vi "trigger test.vi"   [LabVIEW 2012]
uses:
  <vilib>/DAQmx/create/channels.llb/DAQmx Create Channel (AI-Voltage-Basic).vi
  <vilib>/DAQmx/configure/timing.llb/DAQmx Timing (Sample Clock).vi
  <vilib>/DAQmx/configure/trigger.llb/DAQmx Start Trigger (Digital Edge).vi
  <vilib>/DAQmx/write.llb/DAQmx Write (Analog 1D Wfm NChan NSamp).vi
  <vilib>/DAQmx/read.llb/DAQmx Read (Analog 1D DBL 1Chan NSamp).vi
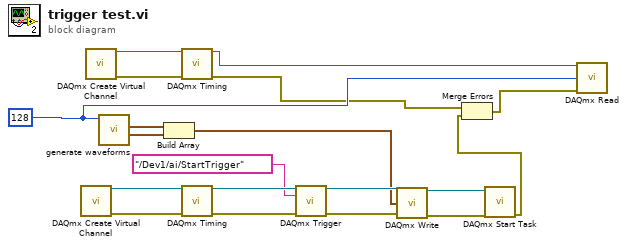
[diagram p0: block diagram]
diagram:
  w6 = 128 ("Number of Samples")
  n1 = call-poly <vilib>:"DAQmx Create Virtual Channel.vi"() -> ("task out"=w18:refnum<k21>, "error out"=w19:errorcluster)  [unwired: 14 in]
  n2 = call-poly <vilib>:"DAQmx Create Virtual Channel.vi"() -> ("task out"=w16:refnum<k21>, "error out"=w17:errorcluster)  [unwired: 14 in]
  n3 = call "generate waveforms.vi"("Number of Samples"=w6) -> ("Y Scan Waveform"=w9:waveform(dbl), "X Scan Waveform"=w8:waveform(dbl))  [unwired: 7 in, 2 out]
  n4 = Build Array(w8, w9) -> (w7:waveform(dbl)[])
  n5 = call-poly <vilib>:"DAQmx Timing.vi"("task/channels in"=w16, "error in"=w17) -> ("task out"=w5:refnum<k21>, "error out"=w3:errorcluster)  [unwired: 12 in]
  n6 = call-poly <vilib>:"DAQmx Timing.vi"("task/channels in"=w18, "error in"=w19) -> ("task out"=w14:refnum<k21>, "error out"=w15:errorcluster)  [unwired: 12 in]
  n7 = call-poly <vilib>:"DAQmx Trigger.vi"("task/channels in"=w14, "source"=tag "/Dev1/ai/StartTrigger", "error in"=w15) -> ("task out"=w11:refnum<k21>, "error out"=w12:errorcluster)  [unwired: 11 in]
  n8 = call-poly <vilib>:"DAQmx Write.vi"("task/channels in"=w11, "data"=w7, "error in"=w12) -> ("task out"=w10:refnum<k21>, "error out"=w4:errorcluster)  [unwired: 10 in, 1 out]
  n9 = call <vilib>:"DAQmx Start Task.vi"("task/channels in"=w10, "error in"=w4) -> ("error out"=w2:errorcluster)  [unwired: 12 in, 1 out]
  n10 = Merge Errors(w3, w2) -> (w1:errorcluster)
  n11 = call-poly <vilib>:"DAQmx Read.vi"("task/channels in"=w5, "number of samples per channel"=w6, "error in"=w1) -> ()  [unwired: 10 in, 3 out]
